vi "Scale Axes.vi"(8 "Axis 3 (throttle)":dbl, 10 "Axis 2 (y)":dbl, 11 "Axis 1 (x)":dbl) -> (2 "Scaled y":dbl, 3 "Scaled x":dbl)   [LabVIEW 2012]
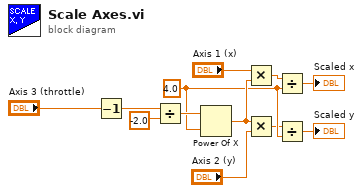
[diagram p0: block diagram]
diagram:
  w5 = 4.0 ("y")
  n1 = Decrement(x="Axis 3 (throttle)") -> (x-1=w11:dbl)
  n2 = Divide(x=w11, y=-2.0) -> (x/y=w9:dbl)
  n3 = Power Of X(1:w5, 2:w9) -> (0:w7:dbl)
  n4 = Multiply(x="Axis 1 (x)", y=w7) -> (x*y=w4:dbl)
  n5 = Multiply(x=w7, y="Axis 2 (y)") -> (x*y=w3:dbl)
  n6 = Divide(x=w4, y=w5) -> (x/y=→"Scaled x":dbl)
  n7 = Divide(x=w3, y=w5) -> (x/y=→"Scaled y":dbl)
